vi "Main.vi"() -> ()   [LabVIEW 2017]
doc: "This Continuous Measurement sample project is based on the Queued Message Handler template.\n\nThe Event Handling Loop generates messages based on user interface actions.\n\nThe Message Handling Loop processes messages generated by the Event Handling Loop, or by other messages. There are also Acquisition and Logging message handling loop subVIs, and a chart updating loop."
uses:
  Settings/Settings.ctl
  Acquisition/Hardware Configuration.ctl
  controls/UI Data.ctl
  controls/UI State.ctl
  <vilib>/Waveform/WDTOps.llb/WDT Index Channel DBL.vi
  <vilib>/measure/matone.llb/Extract Single Tone Information 1 Chan.vi
  <vilib>/measure/mascope.llb/Amplitude and Levels 1 chan.vi
  <vilib>/measure/mascope.llb/Amplitude and Levels N chan.vi
  support/Message Queue/Enqueue Message (Single).vi
  <vilib>/Utility/file.llb/Write Delimited Spreadsheet (DBL).vi
  <vilib>/Utility/file.llb/Write Delimited Spreadsheet (string).vi
  <vilib>/Utility/error.llb/Error Cluster From Error Code.vi
  <vilib>/ErrorRing/Error Ring.xnode
  Acquisition/Acquisition.lvlib
  Settings/Settings.lvlib
  support/User Event - Stop/User Event - Stop.lvlib
  support/Message Queue/Message Queue.lvlib
  <vilib>/measure/NI_MAPro.lvlib
panel:
  out "Reference":waveform(dbl)[](graph)
  out "Channel":waveform(dbl)[](graph)
  in  "Settings":bool
  in  "Start":bool
  in  "Stop":bool
  out "Current":dbl format="%#_4f"
  out "Z":dbl format="%#_4f"
  out "Y":dbl format="%#_4f"
  in  "Component":enum16{"X", "Y", "Z"}(ring)
  out "Diff":cluster{dbl, dbl}(slide)={0.0, -0.043227665706051965} scale=-2.0..2.0
  out "Frequency":dbl format="%#.3f"
  out "X":dbl format="%#_4f"
  out "Target":dbl format="%#_4f"
  out "Input":dbl format="%#_3f"
  out "Settings 2":T1
  out "Status":string
  in  "Exit":bool
  in  "Export":bool
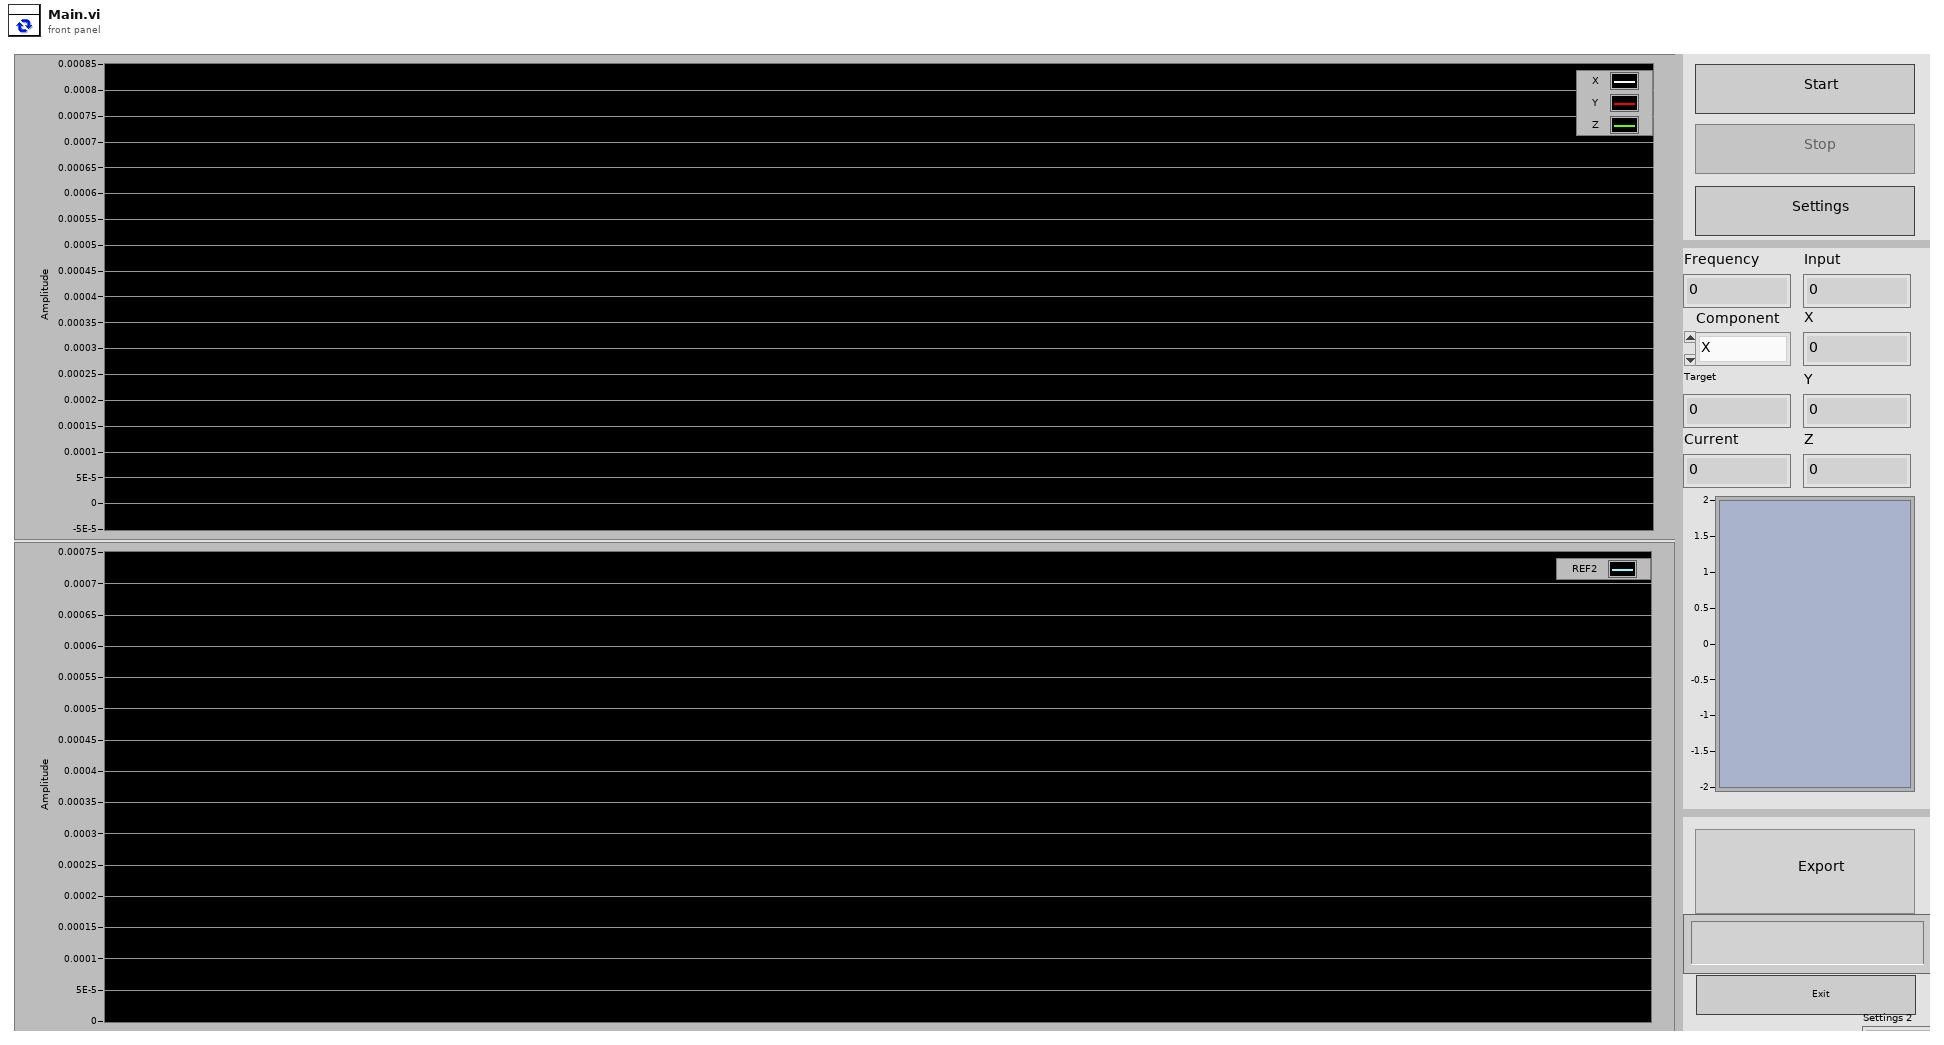
[diagram p1: front panel]
types:
  T1 = typedef "Settings.lvlib/Settings.ctl" = cluster{"Hardware Configuration":T2, "Ga":dbl, "Gv":dbl, "ExportPath":string}
  T2 = typedef "Acquisition.lvlib/Hardware Configuration.ctl" = cluster{"Sensor Channels":tag, "Max Input":dbl, "Min Input":dbl, "Sample Rate":dbl, "DAQmx Task":refnum<k21>, "Reference Channels":tag}
  T3 = typedef "UI State.ctl" = enum16{"Idle", "Acquiring and Logging", "Waiting for Exit", "Waiting for Exit (Acq Stopped)", "Waiting for Stop", "Waiting for Stop (Acq Stopped)"}
  T4 = typedef "UI Data.ctl" = cluster{"Start Ref":refnum<vi>, "Stop Ref":refnum<vi>, "Settings Ref":refnum<vi>, "Status Ref":refnum<vi>, "Exit Ref":refnum<vi>, "Data Ref":refnum<vi>, "Frequency":refnum<vi>, "Input":refnum<vi>, "Target":refnum<vi>, "Current":refnum<vi>, "Diff":refnum<vi>, "Component":refnum<vi>, "X":refnum<vi>, "Y":refnum<vi>, "Z":refnum<vi>}
  T5 = typedef "Message Queue.lvlib/All Message Queues.ctl" = cluster{"UI":refnum<queue>, "Acquisition":refnum<queue>, "Logging":refnum<queue>}
  T6 = enum32{"none", "input signal", "detected signal", "residual signal"}
  T7 = cluster{"method":enum32{"histogram", "peak", "auto select"}, "histogram size":i32, "histogram method":enum16{"mode"}, "reserved":dbl}
  T8 = cluster{"detected frequency":dbl, "amplitude":dbl, "amplitude":dbl, "amplitude":dbl, "amplitude":dbl}
  T9 = cluster{"detected frequency":dbl, "amplitude":dbl, "amplitude":dbl, "amplitude":dbl, "amplitude":dbl}[]
  T10 = enum8{"Enabled", "Disabled", "Disabled and Grayed Out"}
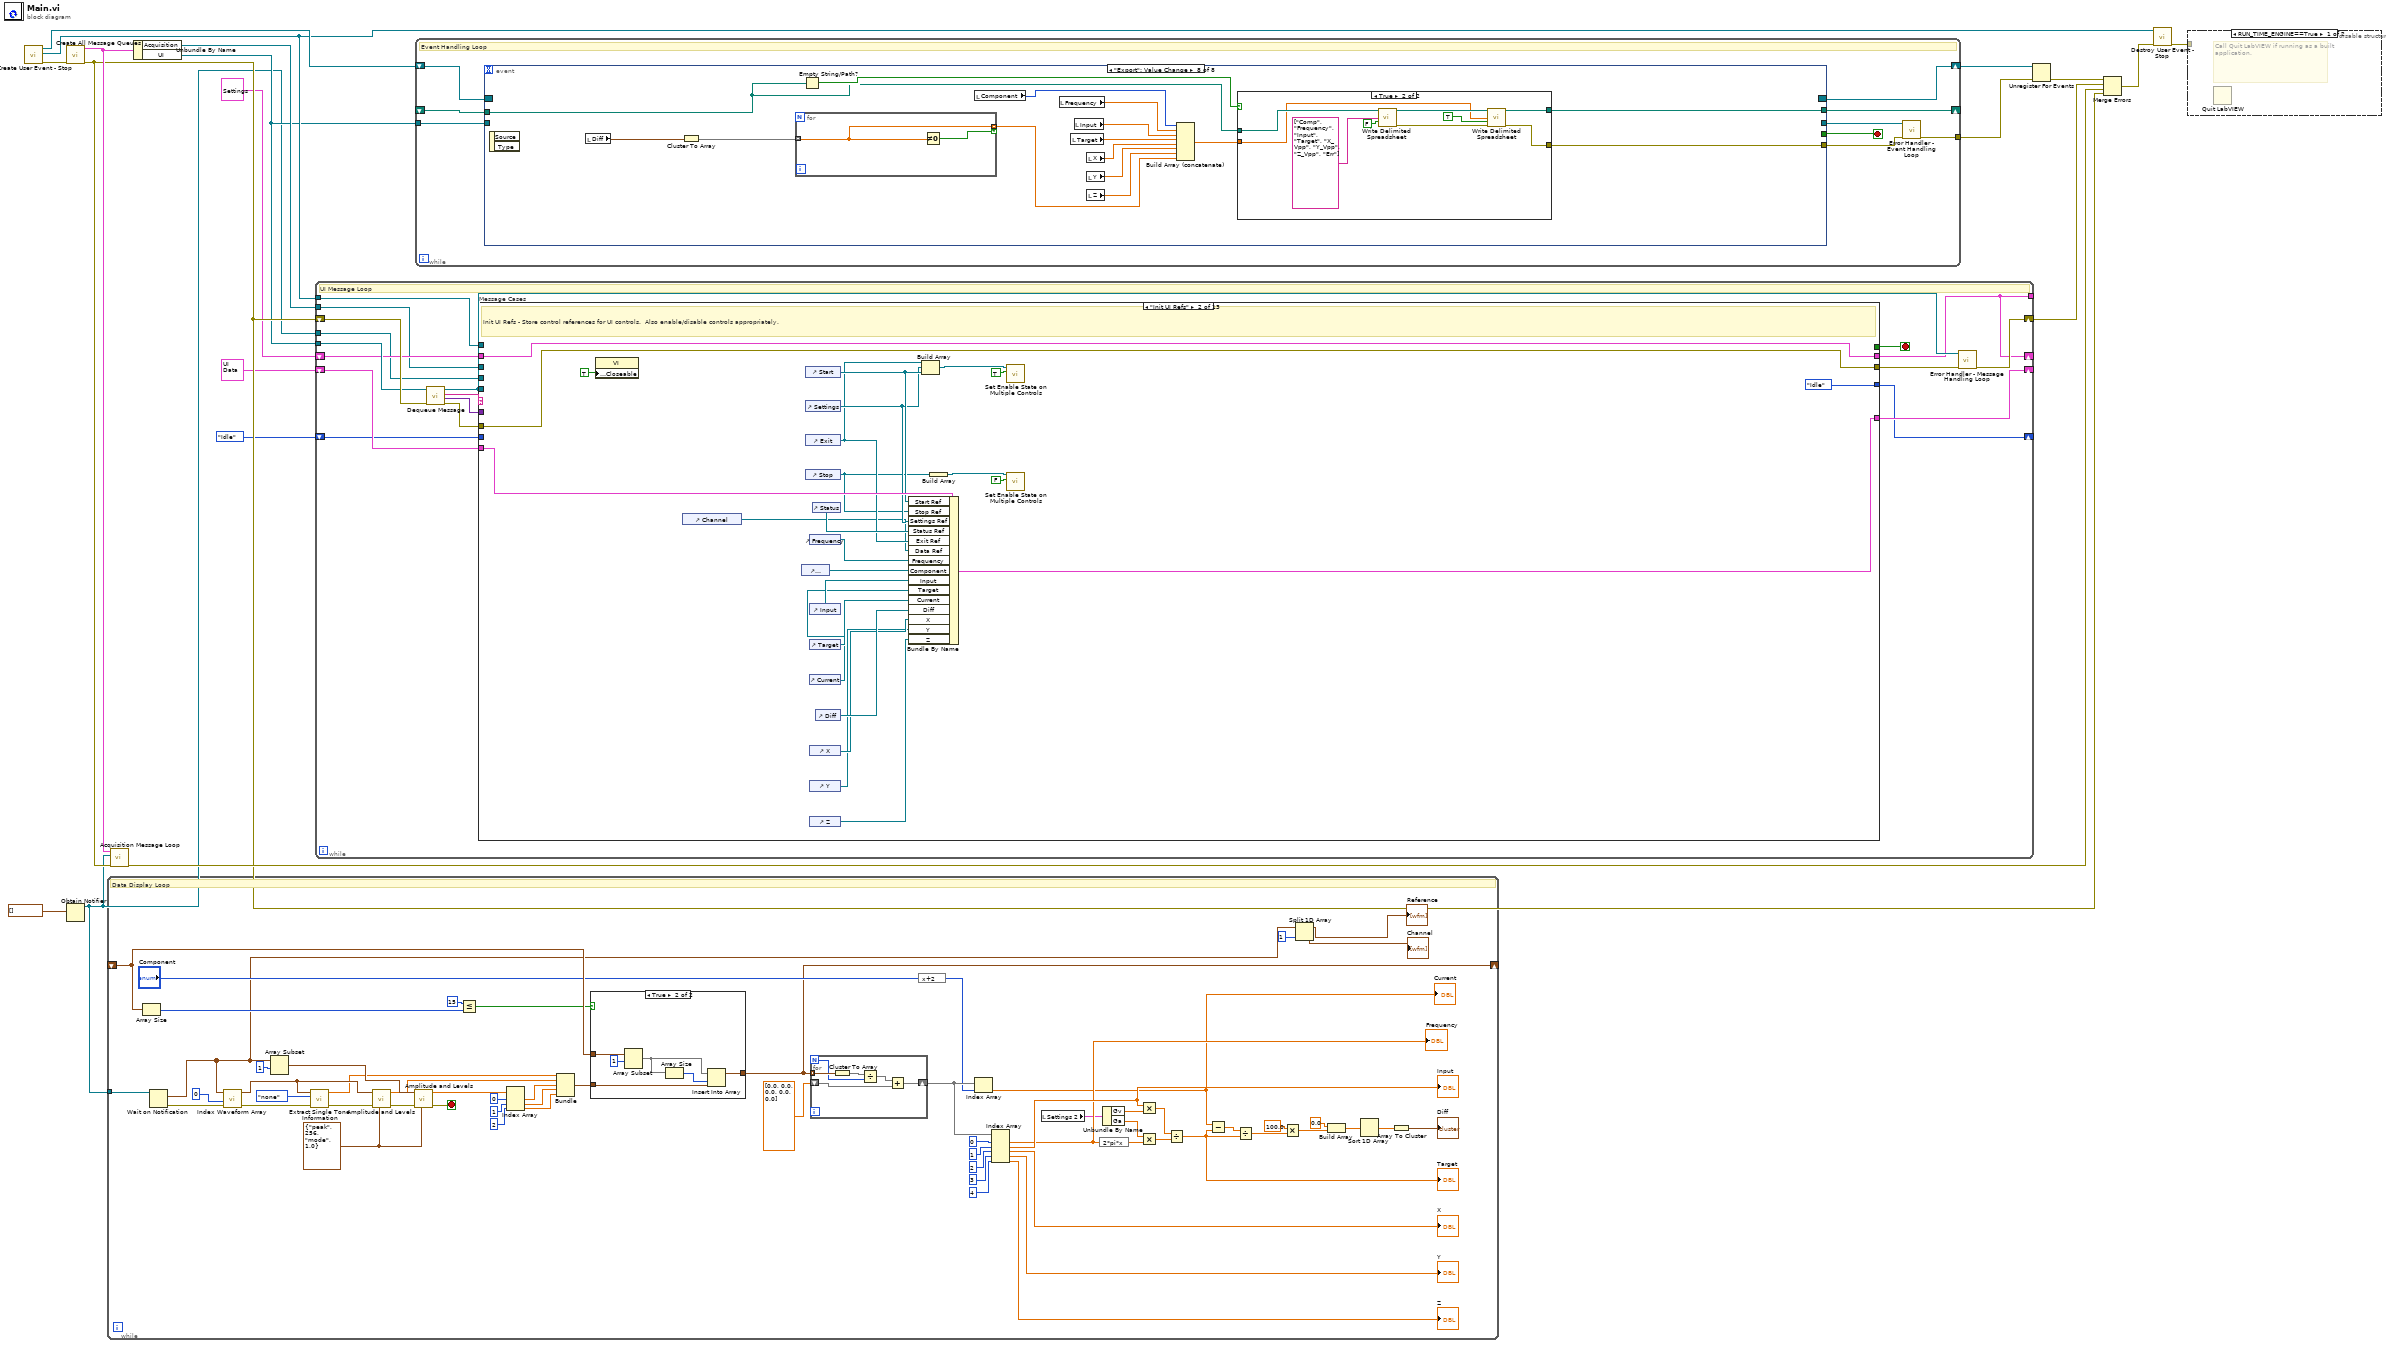
[diagram p0: block diagram]
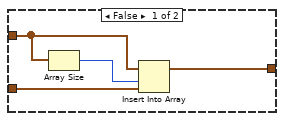
[diagram p3: hidden frame]
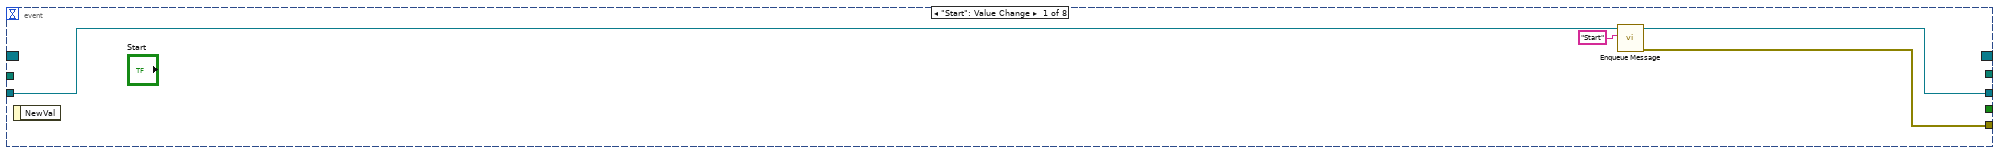
[diagram p4: hidden frame]
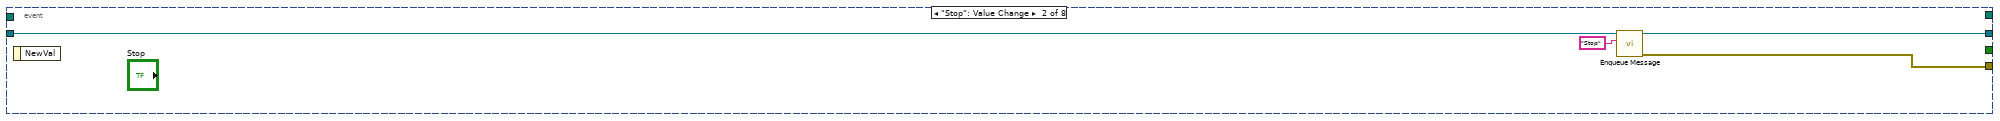
[diagram p5: hidden frame]
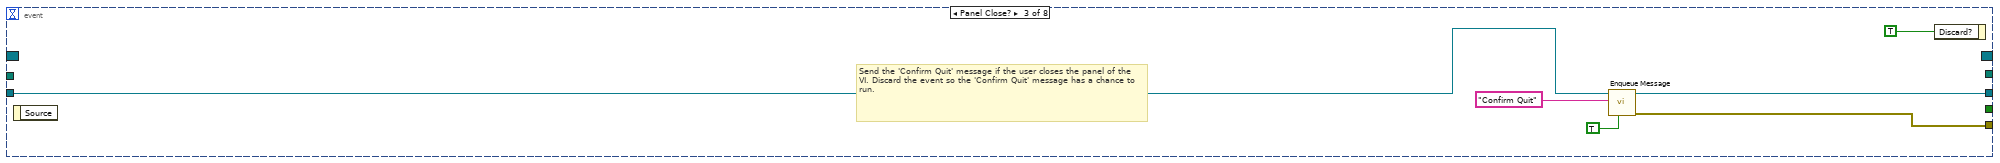
[diagram p6: hidden frame]
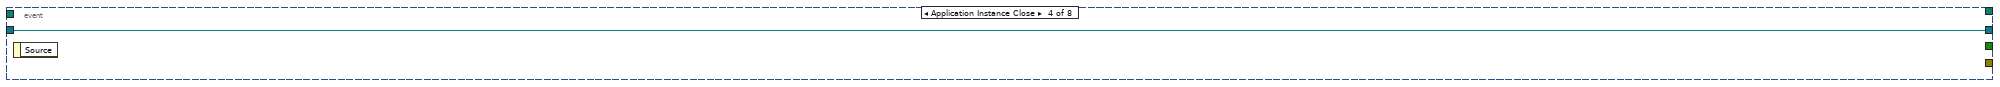
[diagram p7: hidden frame]
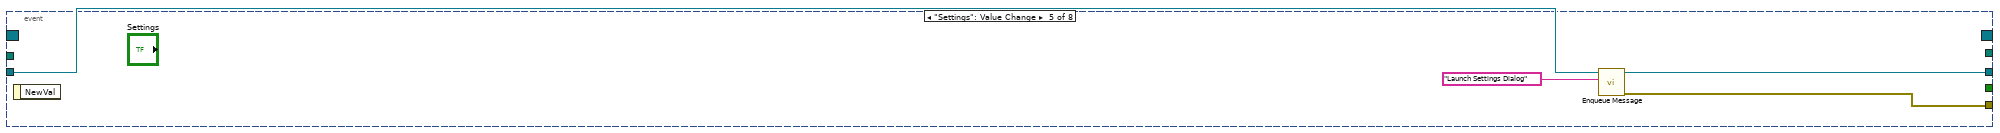
[diagram p8: hidden frame]
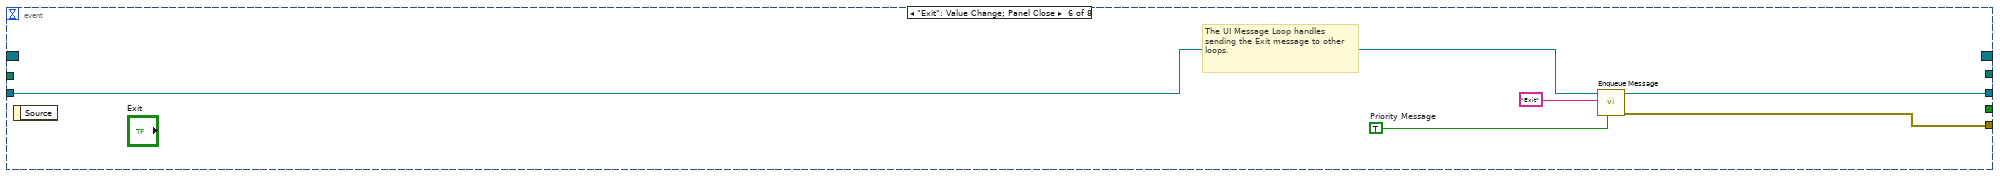
[diagram p9: hidden frame]
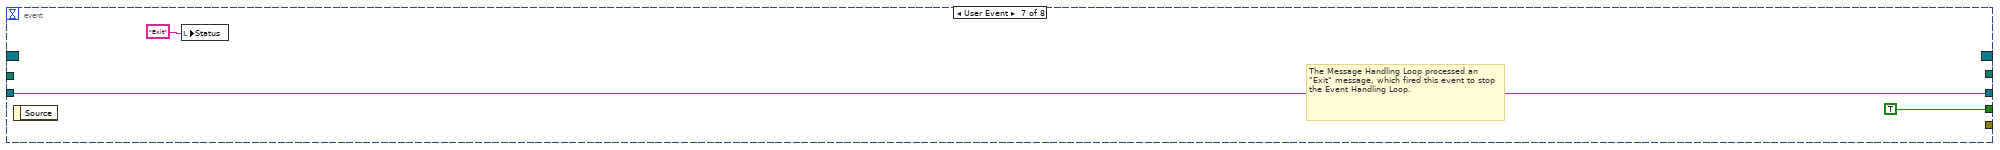
[diagram p10: hidden frame]
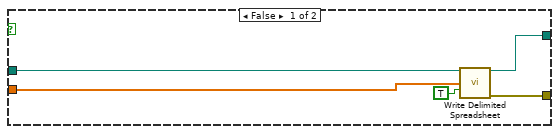
[diagram p11: hidden frame]
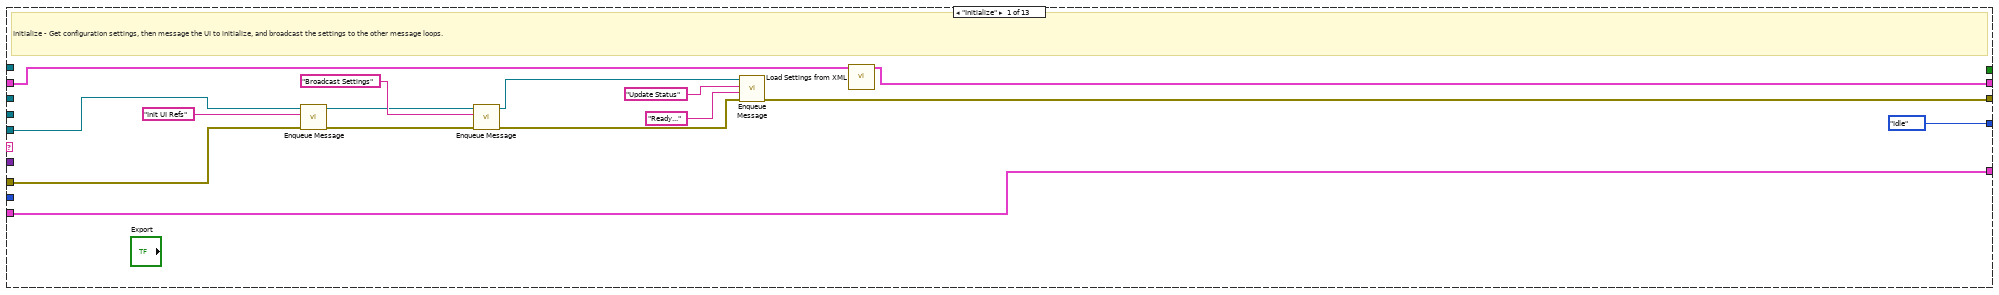
[diagram p12: hidden frame]
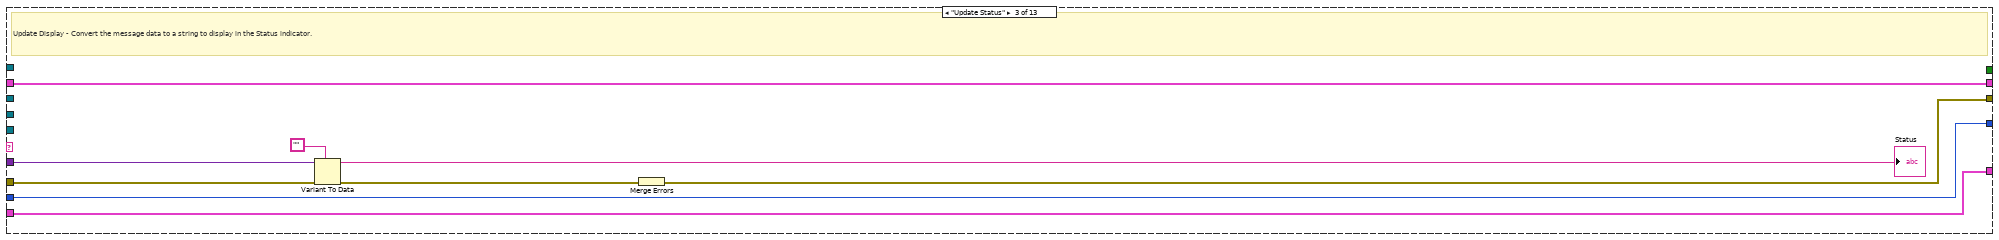
[diagram p13: hidden frame]
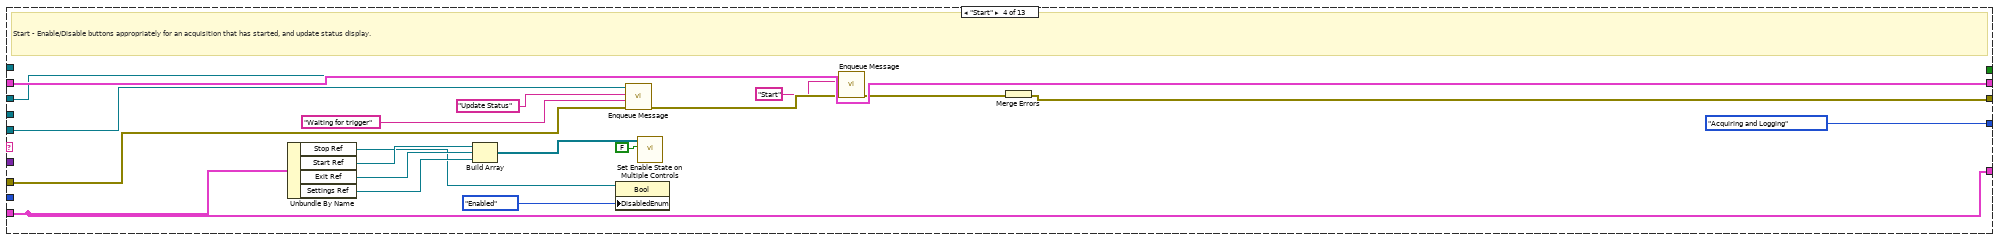
[diagram p14: hidden frame]
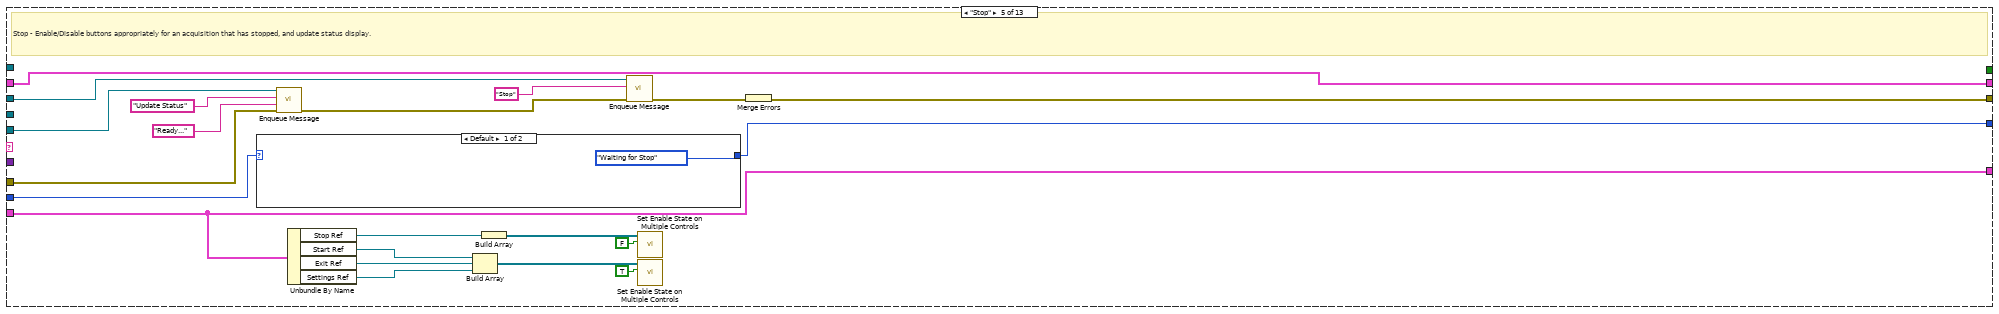
[diagram p15: hidden frame]
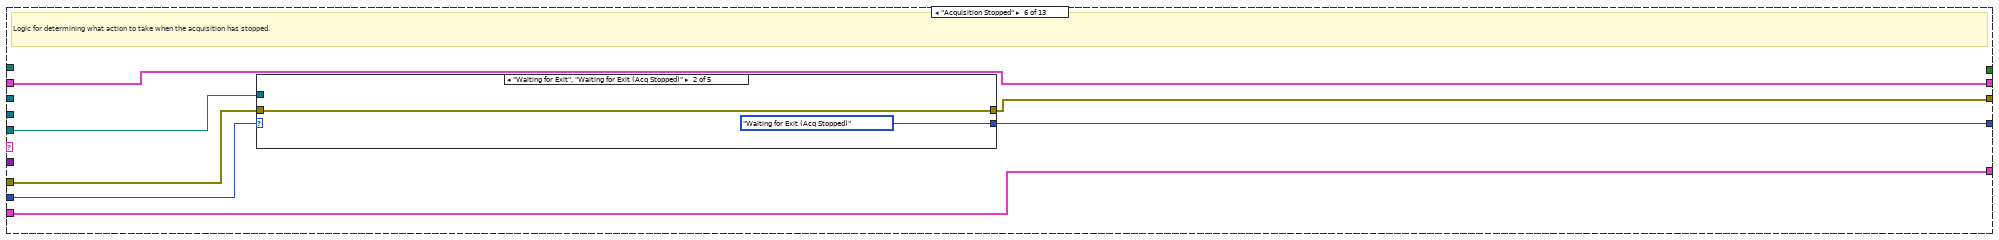
[diagram p17: hidden frame]
diagram:
  n1 = call "Create User Event - Stop.vi"() -> ("error out"=w13:errorcluster, "User Event - Stop"=w15:refnum<user-event>, "Stop Event Registration Refnum"=w16:refnum<event-registration>)  [unwired: 9 in]
  n2 = call "Create All Message Queues.vi"("error in (no error)"=w13) -> ("error out"=w11:errorcluster, "Message Queues out"=w12:T5)  [unwired: 9 in]
  n3 = Obtain Notifier(notification data type=waveform(dbl)[] []) -> (notifier out=w4:refnum<notifier>)  [unwired: 3 in, 2 out]
  n4 = while "Data Display Loop" {
    tunnel: w4 -> [w80]
    shift-right: [w24] -> _
    shift-left: _ -> [w75]
    stop <- w54 stop-if-true
    w52 = T7 {"method"=enum."peak", "histogram size"=256, "histogram method"=enum."mode", "reserved"=1.0} ("state settings")
    # "Data Display Loop"
    n5 = Array Size(array=w75) -> (size(s)=w74:i32)
    n6 = Wait on Notification(notifier=w80) -> (notification=w23:waveform(dbl)[], error out=w77:errorcluster)  [unwired: 3 in, 2 out]
    n7 = call-poly <vilib>:"Index Waveform Array.vi"("error in (no error)"=w77, "index"=0, "waveform array"=w23) -> ("error out"=w76:errorcluster, "waveform"=w35:waveform(dbl))  [unwired: 7 in]
    n8 = Array Subset(array=w23, index=1) -> (w36:waveform(dbl)[])  [unwired: 1 in]
    n9 = call-poly <vilib>:"Extract Single Tone Information.vi"("error in (no error)"=w76, "export mode"=T6."none", "time signal in"=w35) -> ("error out"=w53:errorcluster, "detected frequency"=w34:dbl)  [unwired: 3 in, 4 out]
    n10 = call-poly <vilib>:"Amplitude and Levels.vi"("state settings"=w52, "error in (no error)"=w53, "signal in"=w35) -> ("error out"=w55:errorcluster, "amplitude"=w33:dbl)  [unwired: 5 in, 2 out]
    n11 = call-poly <vilib>:"Amplitude and Levels.vi"("state settings"=w52, "error in (no error)"=w55, "signal(s) in"=w36) -> ("error out"=w54:errorcluster, "amplitude"=w32:dbl[])  [unwired: 5 in, 2 out]
    n12 = Less Or Equal?(x=15, y=w74) -> (x <= y?=w72:bool)
    n13 = Index Array(array=w32, index #1=0 ("index"), index #2=1 ("index"), index #3=2 ("index")) -> (element #1=w28:dbl, element #2=w27:dbl, element #3=w26:dbl)
    n14 = Bundle("detected frequency"=w34, "amplitude"=w33, "amplitude"=w28, "amplitude"=w27, "amplitude"=w26) -> (w25:T8)  [unwired: 1 in]
    n15 = case shown="True" w72 {
      tunnel: w75 -> [w87 w95]
      tunnel: w25 -> [w88 w94]
      tunnel: [w89 w91] -> w24
      frame False {
        n16 = Array Size(array=w87) -> (size(s)=w90:i32)
        n17 = Insert Into Array(array=w87, index=w90, new element=w88) -> (w89:T9)
      }
      frame True {
        n18 = Array Subset(array=w95, index=1) -> (w92:T9)  [unwired: 1 in]
        n19 = Array Size(array=w92) -> (size(s)=w93:i32)
        n20 = Insert Into Array(array=w92, index=w93, new element=w94) -> (w91:T9)
      }
    }
    n21 = for {
      N -> [w85]
      tunnel: w24 -> [w86] mode=indexing
      shift-right: [w82] -> w40
      shift-left: dbl[] [0.0, 0.0, 0.0, 0.0, 0.0] -> [w83]
      n22 = Cluster To Array(cluster=w86) -> (array=w81:dbl[])
      n23 = Divide(x=w81, y=w85) -> (x/y=w84:dbl[])
      n24 = Add(x=w84, y=w83) -> (x+y=w82:dbl[])
    }
    n25 = expression code="x+2"("Component") -> (w39:enum16{"X", "Y", "Z"})
    n26 = Index Array(array=w40, index=w39) -> (element=w38:dbl)
    "Current" <- w38
    n27 = Index Array(array=w40, index #1=0 ("index"), index #2=1 ("index"), index #3=2 ("index"), index #4=3 ("index"), index #5=4 ("index")) -> (element #1=w66:dbl, element #2=w69:dbl, element #3=→"X":dbl, element #4=→"Y":dbl, element #5=→"Z":dbl)
    "Frequency" <- w66
    "Input" <- w69
    n28 = local read "Settings 2"() -> (w59:T1)
    n29 = expression code="2*pi*x"(w66) -> (w65:dbl)
    n30 = Unbundle By Name(w59) -> ("Gv"=w68:dbl, "Ga"=w64:dbl)
    n31 = Multiply(x=w69, y=w68) -> (x*y=w67:dbl)
    n32 = Multiply(x=w64, y=w65) -> (x*y=w63:dbl)
    n33 = Divide(x=w67, y=w63) -> (x/y=w57:dbl)
    "Target" <- w57
    n34 = Subtract(x=w38, y=w57) -> (x-y=w58:dbl)
    n35 = Divide(x=w58, y=w57) -> (x/y=w56:dbl)
    n36 = Multiply(x=100.0, y=w56) -> (x*y=w50:dbl)
    n37 = Split 1D Array(array=w23, index=1) -> (first subarray=→"Reference":waveform(dbl)[], second subarray=→"Channel":waveform(dbl)[])
    n38 = Build Array(0.0 ("element"), w50) -> (w48:dbl[])
    n39 = Sort 1D Array(array=w48) -> (sorted array=w47:dbl[])
    n40 = Array To Cluster(array=w47) -> (cluster=→"Diff":cluster{"[0]":dbl, "[1]":dbl})
  }
  n41 = call "Acquisition Message Loop.vi"("error in (no error)"=w11, "Data Notifier"=w4, "Message Queues"=w12) -> ("error out"=w14:errorcluster)  [unwired: 8 in]
  n42 = Unbundle By Name(w12) -> ("Acquisition"=w7:refnum<queue>, "UI"=w6:refnum<queue>)
  n43 = while {
    tunnel: w6 -> [w108]
    tunnel: w15 -> [w113]
    shift-right: [w101] -> w19
    shift-left: w11 -> [w112]
    shift-right: [w97] -> _
    shift-left: T1 {"Hardware Configuration"={"Sensor Channels"="", "Max Input"=0.0, "Min Input"=0.0, "Sample Rate"=0.0, "DAQmx Task"="", "Reference Channels"=""}, "Ga"=0.0, "Gv"=0.0, "ExportPath"=""} ("Settings") -> [w107]
    shift-right: [w105] -> _
    shift-left: T4 {"Start Ref"=refnum, "Stop Ref"=refnum, "Settings Ref"=refnum, "Status Ref"=refnum, "Exit Ref"=refnum, "Data Ref"=refnum, "Frequency"=refnum, "Input"=refnum, "Target"=refnum, "Current"=refnum, "Diff"=refnum, "Component"=refnum, "X"=refnum, "Y"=refnum, "Z"=refnum} ("Measurement UI Controls") -> [w106]
    tunnel: w7 -> [w104]
    tunnel: w4 -> [w103]
    shift-right: [w98] -> _
    shift-left: UI_State."Idle" ("UI State") -> [w99]
    tunnel: [w97] -> _
    stop <- w114 stop-if-true
    # "UI Message Loop"
    n44 = call "Dequeue Message.vi"("error in (no error)"=w112, "Message Queue"=w108) -> ("error out"=w111:errorcluster, "Message Data"=w109:variant, "Message"=w110:string, "dup Message Queue"=w100:refnum<queue>)  [unwired: 6 in]
    n45 = case "Message Cases" shown="\"Init UI Refs\"" w110 {
      selector: w110 -> [_ _ _ _ _ _ _ _ _ _ _ _ w308]
      tunnel: w100 -> [w119 _ _ w181 w202 w206 _ w237 w252 w262 w292 _ _]
      tunnel: w111 -> [w118 w154 w162 w180 w201 w208 w228 w239 w256 w261 w299 w306 _]
      tunnel: [w125 w154 w163 w182 w203 w207 w231 w234 w247 w260 w300 w305 w309] -> w102
      tunnel: [_ _ _ _ _ _ _ _ _ _ TRUE _ _] -> w114
      tunnel: w109 -> [_ _ w161 _ _ _ _ _ w255 _ _ _ _]
      tunnel: w113 -> [_ _ _ _ _ _ _ _ _ _ w298 _ _]
      tunnel: [w128 w153 w158 w179 w200 w212 w223 w236 w258 w265 w296 w304 w311] -> w97
      tunnel: w107 -> [w129 w153 w158 w179 w200 w212 w223 w240 w258 w265 w296 w304 w311]
      tunnel: w106 -> [w121 w152 w157 w176 w197 w211 w226 w233 w257 w264 w294 w303 w310]
      tunnel: [w121 w151 w157 w176 w197 w211 w226 w233 w257 w264 w294 w303 w310] -> w105
      tunnel: w104 -> [_ _ _ w168 w187 _ w225 _ _ _ w293 _ _]
      tunnel: w103 -> [_ _ _ _ _ _ _ _ _ _ w291 _ _]
      tunnel: w99 -> [_ _ w155 _ w184 w210 w224 w232 w246 w263 _ w302 w307]
      tunnel: [UI_State."Idle" ("UI State") UI_State."Idle" ("UI State") w155 UI_State."Acquiring and Logging" ("UI State") w183 w209 w224 w232 w246 w259 UI_State."Idle" ("UI State") w302 w307] -> w98
      frame "Initialize" {
        # "Initialize - Get configuration settings, then message the UI to initialize, and broadcast the settings to the other message loops."
        n46 = call-poly "Enqueue Message.vi"("error in (no error)"=w118, "Message"="Init UI Refs", "Message Queue"=w119) -> ("error out"=w116:errorcluster, "dup Message Queue"=w117:refnum<queue>)  [unwired: 7 in]
        n47 = call-poly "Enqueue Message.vi"("error in (no error)"=w116, "Message"="Broadcast Settings", "Message Queue"=w117) -> ("error out"=w127:errorcluster, "dup Message Queue"=w126:refnum<queue>)  [unwired: 7 in]
        n48 = call-poly "Enqueue Message.vi"("error in (no error)"=w127, "Message Data"="Ready..." ("Ready..."), "Message"="Update Status", "Message Queue"=w126) -> ("error out"=w125:errorcluster)  [unwired: 6 in, 1 out]
        n49 = call "Load Settings from XML.vi"("Settings in"=w129) -> ("Settings out"=w128:T1)  [unwired: 9 in, 1 out]
      }
      frame "Init UI Refs" {
        # "Init UI Refs - Store control references for UI controls.  Also enable/disable controls appropriately."
        n50 = property class="VI"("Front Panel.Closeable"=TRUE ("Front Panel Window:Closeable")) -> ()  [unwired: 2 in, 2 out]
        n51 = control-ref of="Channel"() -> (w139:refnum<vi>)
        n52 = control-ref of="Component"() -> (w134:refnum<vi>)
        n53 = control-ref of="Start"() -> (w147:refnum<vi>)
        n54 = control-ref of="Settings"() -> (w144:refnum<vi>)
        n55 = control-ref of="Exit"() -> (w143:refnum<vi>)
        n56 = control-ref of="Stop"() -> (w142:refnum<vi>)
        n57 = control-ref of="Frequency"() -> (w138:refnum<vi>)
        n58 = control-ref of="Input"() -> (w137:refnum<vi>)
        n59 = control-ref of="Target"() -> (w136:refnum<vi>)
        n60 = control-ref of="Current"() -> (w130:refnum<vi>)
        n61 = control-ref of="X"() -> (w133:refnum<vi>)
        n62 = control-ref of="Y"() -> (w132:refnum<vi>)
        n63 = control-ref of="Z"() -> (w131:refnum<vi>)
        n64 = control-ref of="Status"() -> (w148:refnum<vi>)
        n65 = control-ref of="Diff"() -> (w135:refnum<vi>)
        n66 = Bundle By Name(cluster=w152, "Start Ref"=w147, "Stop Ref"=w142, "Settings Ref"=w144, "Status Ref"=w148, "Exit Ref"=w143, "Data Ref"=w139, "Frequency"=w138, "Component"=w134, "Input"=w137, "Target"=w136, "Current"=w130, "Diff"=w135, "X"=w133, "Y"=w132, "Z"=w131) -> (w151:T4)
        n67 = Build Array(w143, w144, w147) -> (w146:refnum<vi>[])
        n68 = Build Array(w142) -> (w141:refnum<vi>[])
        n69 = call "Set Enable State on Multiple Controls.vi"("Enable?"=TRUE, "Controls"=w146) -> ()  [unwired: 10 in]
        n70 = call "Set Enable State on Multiple Controls.vi"("Enable?"=FALSE, "Controls"=w141) -> ()  [unwired: 10 in]
      }
      frame "Update Status" {
        # "Update Display - Convert the message data to a string to display in the Status indicator."
        n71 = Variant To Data(error in=w162, type="", Variant=w161) -> (data=→"Status":string, error out=w159:errorcluster)
        n72 = Merge Errors(w159) -> (w163:errorcluster)
      }
      frame "Start" {
        # "Start - Enable/Disable buttons appropriately for an acquisition that has started, and update status display."
        n73 = Unbundle By Name(w176) -> ("Stop Ref"=w165:refnum<vi>, "Start Ref"=w173:refnum<vi>, "Exit Ref"=w172:refnum<vi>, "Settings Ref"=w171:refnum<vi>)
        n74 = Build Array(w173, w172, w171) -> (w174:refnum<vi>[])
        n75 = property class="Bool"(reference=w165, "DisabledEnum"=T10."Enabled" ("Disabled")) -> ()  [unwired: 1 in, 2 out]
        n76 = call-poly "Enqueue Message.vi"("error in (no error)"=w180, "Message Data"="Waiting for trigger" ("Waiting for trigger"), "Message"="Update Status", "Message Queue"=w181) -> ("error out"=w170:errorcluster)  [unwired: 6 in, 1 out]
        n77 = call "Set Enable State on Multiple Controls.vi"("Enable?"=FALSE, "Controls"=w174) -> ()  [unwired: 10 in]
        n78 = call-poly "Enqueue Message.vi"("error in (no error)"=w170, "Message"="Start", "Message Queue"=w168) -> ("error out"=w169:errorcluster)  [unwired: 7 in, 1 out]
        n79 = Merge Errors(w169) -> (w182:errorcluster)
      }
      frame "Stop" {
        # "Stop - Enable/Disable buttons appropriately for an acquisition that has stopped, and update status display."
        n80 = case shown="Default" w184 {
          selector: w184 -> [_ w205]
          tunnel: [UI_State."Waiting for Stop" ("UI State") w205] -> w183
          frame Default {
          }
          frame "Waiting for Exit" {
          }
        }
        n81 = call-poly "Enqueue Message.vi"("error in (no error)"=w201, "Message Data"="Ready..." ("Ready..."), "Message"="Update Status", "Message Queue"=w202) -> ("error out"=w189:errorcluster)  [unwired: 6 in, 1 out]
        n82 = Unbundle By Name(w197) -> ("Stop Ref"=w185:refnum<vi>, "Start Ref"=w192:refnum<vi>, "Exit Ref"=w191:refnum<vi>, "Settings Ref"=w190:refnum<vi>)
        n83 = Build Array(w192, w191, w190) -> (w195:refnum<vi>[])
        n84 = Build Array(w185) -> (w194:refnum<vi>[])
        n85 = call-poly "Enqueue Message.vi"("error in (no error)"=w189, "Message"="Stop", "Message Queue"=w187) -> ("error out"=w188:errorcluster)  [unwired: 7 in, 1 out]
        n86 = call "Set Enable State on Multiple Controls.vi"("Enable?"=FALSE, "Controls"=w194) -> ()  [unwired: 10 in]
        n87 = call "Set Enable State on Multiple Controls.vi"("Enable?"=TRUE, "Controls"=w195) -> ()  [unwired: 10 in]
        n88 = Merge Errors(w188) -> (w203:errorcluster)
      }
      frame "Acquisition Stopped" {
        # "Logic for determining what action to take when the acquisition has stopped."
        n89 = case shown="\"Waiting for Exit\", \"Waiting for Exit (Acq Stopped)\"" w210 {
          selector: w210 -> [w214 _ w218 w219 _]
          tunnel: [w214 UI_State."Waiting for Exit (Acq Stopped)" ("UI State") w218 w219 UI_State."Waiting for Stop (Acq Stopped)" ("UI State")] -> w209
          tunnel: w208 -> [w213 w215 w217 w220 w221]
          tunnel: [w213 w215 w217 w220 w221] -> w207
          tunnel: w206 -> [_ _ _ _ _]
          frame Default {
          }
          frame "Waiting for Exit", "Waiting for Exit (Acq Stopped)" {
          }
          frame "Acquiring and Logging" {
          }
          frame "Idle" {
          }
          frame "Waiting for Stop (Acq Stopped)" {
          }
        }
      }
      frame "Broadcast settings" {
        # "Send the 'Update Settings' message to the Logging and Acquisition message loops."
        n90 = Unbundle By Name(w223) -> ("Hardware Configuration"=w229:T2)
        n91 = call-poly "Enqueue Message.vi"("Message Data"=w229, "Message"="Update Settings", "Message Queue"=w225) -> ("error out"=w230:errorcluster)  [unwired: 7 in, 1 out]
        n92 = Merge Errors(w230, w228) -> (w231:errorcluster)
        "Settings 2" <- w223
      }
      frame "Launch Settings Dialog" {
        # "Launch the Settings Dialog when the user clicks the 'Settings' button."
        n93 = call "Settings Dialog.vi"("error in (no error)"=w239, "Settings in"=w240) -> ("error out"=w235:errorcluster, "Cancelled?"=w238:bool, "Settings out"=w236:T1)  [unwired: 6 in, 1 out]
        n94 = case shown="False" w238 {
          tunnel: w237 -> [w244 _]
          tunnel: w235 -> [w243 w245]
          tunnel: [w242 w245] -> w234
          frame False {
            n95 = call-poly "Enqueue Message.vi"("error in (no error)"=w243, "Message"="Broadcast Settings", "Message Queue"=w244) -> ("error out"=w242:errorcluster)  [unwired: 7 in, 1 out]
          }
          frame True {
          }
        }
      }
      frame "Error" {
        # "Error - Check the error message data and respond accordingly. This message is sent by the \"Error Handler\" VIs at the end of each loop in this application."
        n96 = Variant To Data(error in=w256, type=errorcluster {"status"=FALSE, "code"=0, "source"=""} ("error out"), Variant=w255) -> (data=w253:errorcluster, error out=w249:errorcluster)
        n97 = call <vilib>:"Simple Error Handler.vi"("error in (no error)"=w253) -> ()  [unwired: 4 in, 5 out]
        n98 = call-poly "Enqueue Message.vi"("Priority Message? (F)"=TRUE, "Message"="Exit", "Message Queue"=w252) -> ("error out"=w248:errorcluster)  [unwired: 7 in, 1 out]
        n99 = Merge Errors(w248, w249) -> (w247:errorcluster)
      }
      frame "Confirm Quit" {
        # "Confirm Quit - Message that can confirm whether or not the user wants to exit the application."
        n100 = case shown="\"Acquiring and Logging\"" w263 {
          tunnel: w262 -> [w270 w276]
          tunnel: w261 -> [w269 w274]
          tunnel: [w266 w273] -> w260
          tunnel: [UI_State."Idle" ("UI State") w272] -> w259
          frame Default {
            n101 = call-poly "Enqueue Message.vi"("Priority Message? (F)"=TRUE, "error in (no error)"=w269, "Message"="Exit", "Message Queue"=w270) -> ("error out"=w266:errorcluster)  [unwired: 6 in, 1 out]
          }
          frame "Acquiring and Logging" {
            n102 = Two Button Dialog(message="Are you sure you want to quit while the acquisition is running?" ("Confirm Quit Message"), 1:"No" ("No"), 2:"Yes" ("Yes")) -> (T button?=w275:bool)
            n103 = case shown="True" w275 {
              tunnel: w276 -> [_ w286]
              tunnel: w274 -> [w280 w285]
              tunnel: [w280 w284] -> w273
              tunnel: [UI_State."Acquiring and Logging" ("UI State") UI_State."Waiting for Exit" ("UI State")] -> w272
              frame False {
                # "User did not want to quit."
              }
              frame True {
                n104 = call-poly "Enqueue Message.vi"("error in (no error)"=w285, "Message"="Stop", "Message Queue"=w286) -> ("error out"=w284:errorcluster)  [unwired: 7 in, 1 out]
              }
            }
          }
        }
      }
      frame "Exit" {
        # "Exit - Fire the User Event to stop the Event Handling Loop.  Also send Exit messages to the Acquisition and Logging loops."
        n105 = call-poly "Enqueue Message.vi"("Priority Message? (F)"=TRUE, "Message"="Exit", "Message Queue"=w293) -> ()  [unwired: 7 in, 2 out]
        n106 = Release Queue(queue=w292, error in (no error)=w299) -> (error out=w290:errorcluster)  [unwired: 1 in, 2 out]
        n107 = Release Notifier(notifier=w291, error in (no error)=w290) -> (error out=w289:errorcluster)  [unwired: 1 in, 2 out]
        n108 = call "Fire User Event - Stop.vi"("User Event - Stop"=w298) -> ("error out"=w297:errorcluster)  [unwired: 10 in]
        n109 = Merge Errors(w297, w289) -> (w300:errorcluster)
      }
      frame "---Copy This Frame---" {
        # "Duplicate this frame when creating new messages.  Change this comment in the duplicated frame to describe this message."
        n110 = Merge Errors(w306) -> (w305:errorcluster)
      }
      frame Default {
        # "'Default' case only runs if there is a message that isn't defined in any of the other cases.  Output a programming error."
        n111 = xnode "Error Ring"("parameter 0"=w308) -> ("error out"=w309:errorcluster)
      }
    }
    n112 = call "Error Handler - Message Handling Loop.vi"("error in (no error)"=w102, "Message Queue"=w100) -> ("dup error in"=w101:errorcluster)  [unwired: 8 in, 1 out]
  }
  n113 = while {
    tunnel: w6 -> [w326]
    tunnel: [w321] -> w18
    shift-right: [w325] -> w9
    shift-left: w16 -> [w327]
    shift-right: [w319] -> _
    shift-left: _ -> [w320]
    stop <- w324 stop-if-true
    # "Event Handling Loop"
    n114 = event shown="[7] \"Export\": Value Change" {
      selector: w327 -> [_ _ _ _ _ _ _ _]
      dyn-events: [_ _ _ _ _ _ _ _] -> w325
      timeout: _ -> [_ _ _ _ _ _ _ _]
      tunnel: [_ _ _ _ _ _ TRUE ("Discard?") _] -> w324
      tunnel: w326 -> [w329 w334 w341 w342 w344 w348 w352 _]
      tunnel: [w331 w333 w336 _ w346 w351 _ w368] -> w322
      tunnel: [w328 w332 w337 w342 w343 w347 w352 _] -> w323
      tunnel: w320 -> [_ _ _ _ _ _ _ w366]
      tunnel: [_ _ _ _ _ _ _ w369] -> w319
      event "Start": Value Change {
        n115 = event-data() -> ()  [unwired: 1 in, 1 out]
        n116 = call-poly "Enqueue Message.vi"("Message"="Start", "Message Queue"=w329) -> ("error out"=w331:errorcluster, "dup Message Queue"=w328:refnum<queue>)  [unwired: 8 in]
      }
      event "Stop": Value Change {
        n117 = event-data() -> ()  [unwired: 1 in, 1 out]
        n118 = call-poly "Enqueue Message.vi"("Message"="Stop", "Message Queue"=w334) -> ("error out"=w333:errorcluster, "dup Message Queue"=w332:refnum<queue>)  [unwired: 8 in]
      }
      event Panel Close? {
        # "Send the 'Confirm Quit' message if the user closes the panel of the VI. Discard the event so the 'Confirm Quit' message has a chance to run."
        n119 = event-data() -> ()  [unwired: 1 in, 1 out]
        n120 = call-poly "Enqueue Message.vi"("Priority Message? (F)"=TRUE, "Message"="Confirm Quit", "Message Queue"=w341) -> ("error out"=w336:errorcluster, "dup Message Queue"=w337:refnum<queue>)  [unwired: 7 in]
        n121 = event-data("Discard?"=TRUE) -> ()  [unwired: 1 in, 1 out]
      }
      event Application Instance Close {
        n122 = event-data() -> ()  [unwired: 1 in, 1 out]
      }
      event "Settings": Value Change {
        n123 = event-data() -> ()  [unwired: 1 in, 1 out]
        n124 = call-poly "Enqueue Message.vi"("Message"="Launch Settings Dialog", "Message Queue"=w344) -> ("error out"=w346:errorcluster, "dup Message Queue"=w343:refnum<queue>)  [unwired: 8 in]
      }
      event "Exit": Value Change; Panel Close {
        w349 = TRUE  # Priority Message
        # "The UI Message Loop handles sending the Exit message to other loops."
        n125 = event-data() -> ()  [unwired: 1 in, 1 out]
        n126 = call-poly "Enqueue Message.vi"("Priority Message? (F)"=w349, "Message"="Exit", "Message Queue"=w348) -> ("error out"=w351:errorcluster, "dup Message Queue"=w347:refnum<queue>)  [unwired: 7 in]
      }
      event User Event {
        # "The Message Handling Loop processed an \"Exit\" message, which fired this event to stop the Event Handling Loop."
        n127 = event-data() -> ()  [unwired: 1 in, 1 out]
        n128 = local write "Status"("Exit" ("Exit String")) -> ()
      }
      event "Export": Value Change {
        n129 = event-data() -> ()  [unwired: 1 in, 2 out]
        n130 = local read "Diff"() -> (w361:cluster{dbl, dbl})
        n131 = Cluster To Array(cluster=w361) -> (array=w362:dbl[])
        n132 = for {
          tunnel: w362 -> [w371] mode=indexing
          tunnel: [w371] -> w365 mode=indexing if=w370
          n133 = Not Equal To 0?(x=w371) -> (x != 0?=w370:bool)
        }
        n134 = Empty String/Path?(string/path=w366) -> (empty?=w367:bool)
        n135 = local read "Component"() -> (w356:enum16{"X", "Y", "Z"})
        n136 = local read "Frequency"() -> (w357:dbl)
        n137 = local read "Target"() -> (w359:dbl)
        n138 = local read "Input"() -> (w358:dbl)
        n139 = local read "X"() -> (w360:dbl)
        n140 = local read "Y"() -> (w363:dbl)
        n141 = local read "Z"() -> (w364:dbl)
        n142 = Build Array (concatenate)(w356, w357, w358, w359, w360, w363, w364, w365) -> (w355:dbl[])
        n143 = case shown="True" w367 {
          tunnel: w366 -> [w376 w385]
          tunnel: [w375 w381] -> w369
          tunnel: [w373 w380] -> w368
          tunnel: w355 -> [w372 w378]
          frame False {
            n144 = call-poly <vilib>:"Write Delimited Spreadsheet.vi"("file path (dialog if empty)"=w376, "1D data"=w372, "append to file? (new file:F)"=TRUE) -> ("new file path (Not A Path if cancelled)"=w375:path, "error out"=w373:errorcluster)  [unwired: 11 in]
          }
          frame True {
            n145 = call-poly <vilib>:"Write Delimited Spreadsheet.vi"("file path (dialog if empty)"=w385, "1D data"=string[] ["Comp", "Frequency", "Input", "Target", "X_Vpp", "Y_Vpp", "Z_Vpp", "Err"], "append to file? (new file:F)"=FALSE) -> ("new file path (Not A Path if cancelled)"=w382:path, "error out"=w383:errorcluster)  [unwired: 11 in]
            n146 = call-poly <vilib>:"Write Delimited Spreadsheet.vi"("file path (dialog if empty)"=w382, "1D data"=w378, "append to file? (new file:F)"=TRUE, "error in (no error)"=w383) -> ("new file path (Not A Path if cancelled)"=w381:path, "error out"=w380:errorcluster)  [unwired: 10 in]
          }
        }
      }
    }
    n147 = call "Error Handler - Event Handling Loop.vi"("error in (no error)"=w322, "Message Queue"=w323) -> ("dup error in"=w321:errorcluster)  [unwired: 8 in, 1 out]
  }
  n148 = Unregister For Events(event registration refnum=w9, error in=w18) -> (error out=w10:errorcluster)
  n149 = Merge Errors(w10, w19, w14, w11) -> (w17:errorcluster)
  n150 = call "Destroy User Event - Stop.vi"("error in (no error)"=w17, "User Event - Stop"=w15) -> ("error out"=w3:errorcluster)  [unwired: 9 in]
  n151 = disable-structure shown="RUN_TIME_ENGINE==True" {
    disable-tunnel: w3 -> [_ _]
    frame condition #0 {
      # "Call Quit LabVIEW if running as a built application."
      n152 = Quit LabVIEW() -> ()  [unwired: 1 in]
    }
    frame condition #1 (active) {
    }
  }
